vi "Create Session.vi"(8 "error in (no error)":errorcluster, 11 "Session Id":u64) -> (0 "error out":errorcluster, 1 "Run Time Configuration":string, 2 "Edit Time Configuration":string, 3 "Session out":refnum<class "Plugin Session.lvclass">, 4 "Panel Size":T1)   [LabVIEW 2021, in "InstrumentStudio Plugin SDK.lvlib" / "Plugin Session.lvclass"]
doc: "Call this VI with the Session Id as the first SDK call at the beginning of your plugin VI. This VI sets up the events and other data needed for the plugin panel and framework to communicate. If you need to know the panel size for your plugin panel to adjust its front panel, this VI will return the size. Some plugin panels support both large and small panel sizes and need to adjust the visuals on their front panel to better fit into that panel size. LabVIEW plugin panels are uniquely identified by the Plugin Session which is set by the framework when the plugin is run. Plugins must have a control named 'Session Id' which is a U64 numeric control on their plugin VI front panel so the framework can correctly set it. This 'Session Id' is then passed to Create Session.vi to begin the plugin session. This control can be placed on the user's VI by right-clicking on the input of the Create Session.vi and choosing 'Create Control'.\nThe Plugin Session returned is then used to call other SDK VIs during execution of the plugin VI to get or set properties of the plugin panel or to notify the framework of various events."
uses:
  Plugin Session.lvclass
  Panel Size.ctl
  Plugin Events.ctl
  Event Registration Refnum.ctl
  Plugin Session.lvclass/Plugin Session.ctl
  Read Edit Time Configuration.vi
  Read Run Time Configuration.vi
  InstrumentStudio Plugin SDK.lvlib
  NationalInstruments.VIHost.Interop.dll
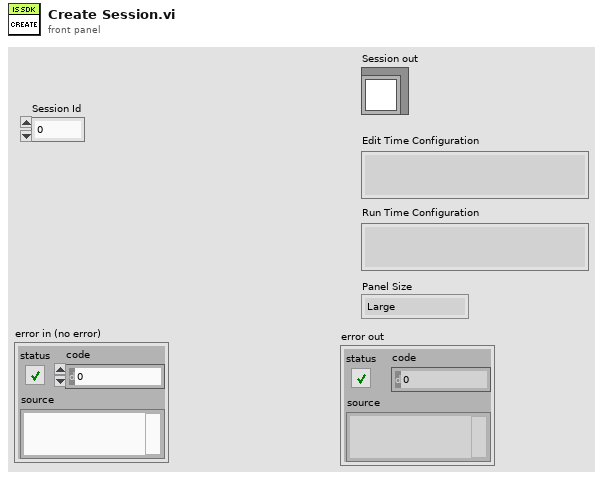
[diagram p1: front panel]
types:
  T1 = typedef "InstrumentStudio Plugin SDK.lvlib/Panel Size.ctl" = enum32{"Large", "Small"}
  T2 = typedef "InstrumentStudio Plugin SDK.lvlib/Plugin Events.ctl" = cluster{"Shutdown":refnum<user-event>, "Project Saved":refnum<user-event>, "Stop All Outputs":refnum<user-event>, "Generic Message":refnum<user-event>}
  T3 = typedef "InstrumentStudio Plugin SDK.lvlib/Event Registration Refnum.ctl" = refnum<event-registration>
  T4 = cluster{"Session Id":u64, "Plugin Events":T2, "Event Refnum":T3}
  T5 = cluster{"Name":string, "Data":string, "Completion Id":i64}
  T6 = cluster{"Project Path":path, "Completion Id":i64}
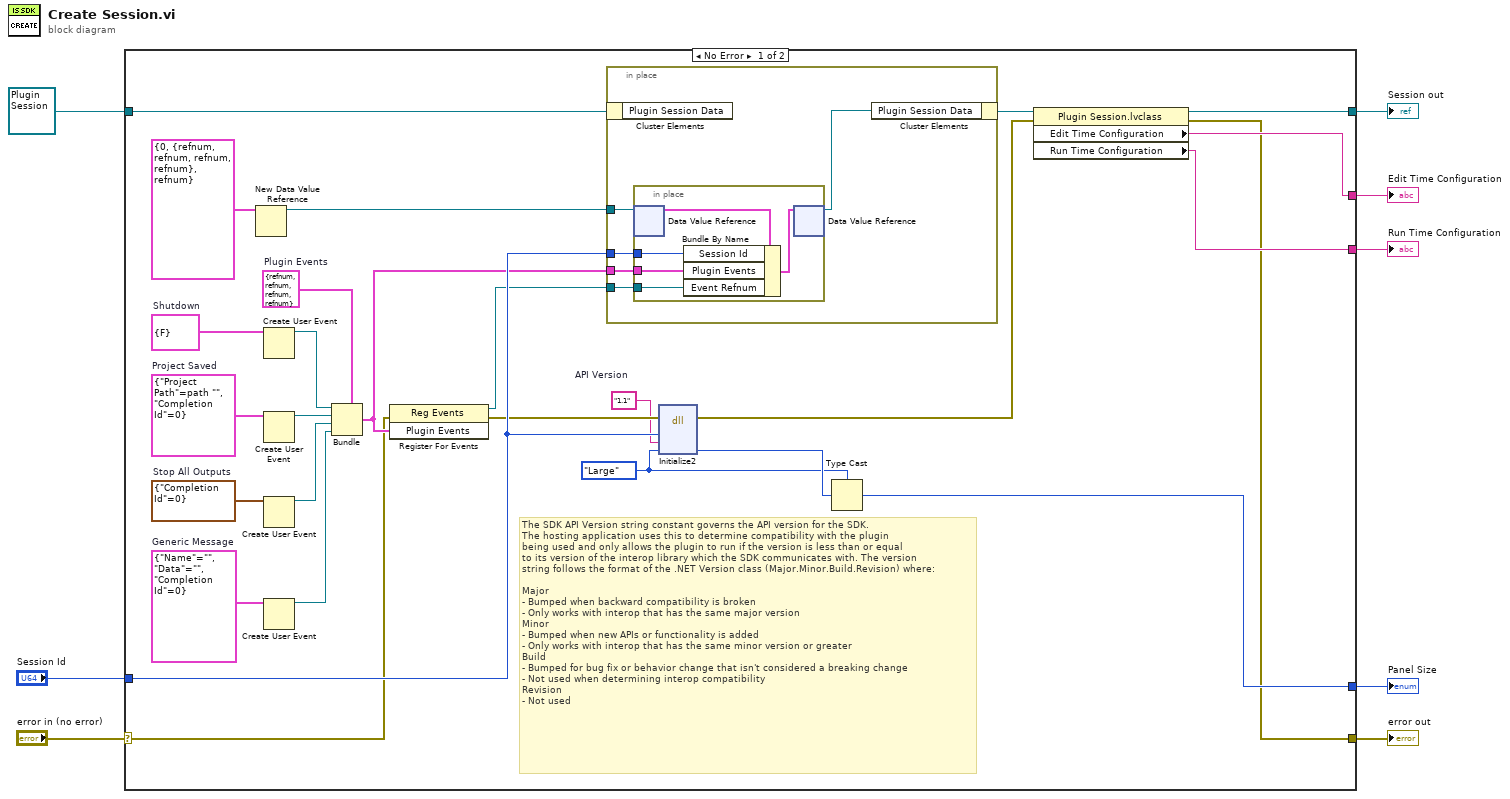
[diagram p0: block diagram]
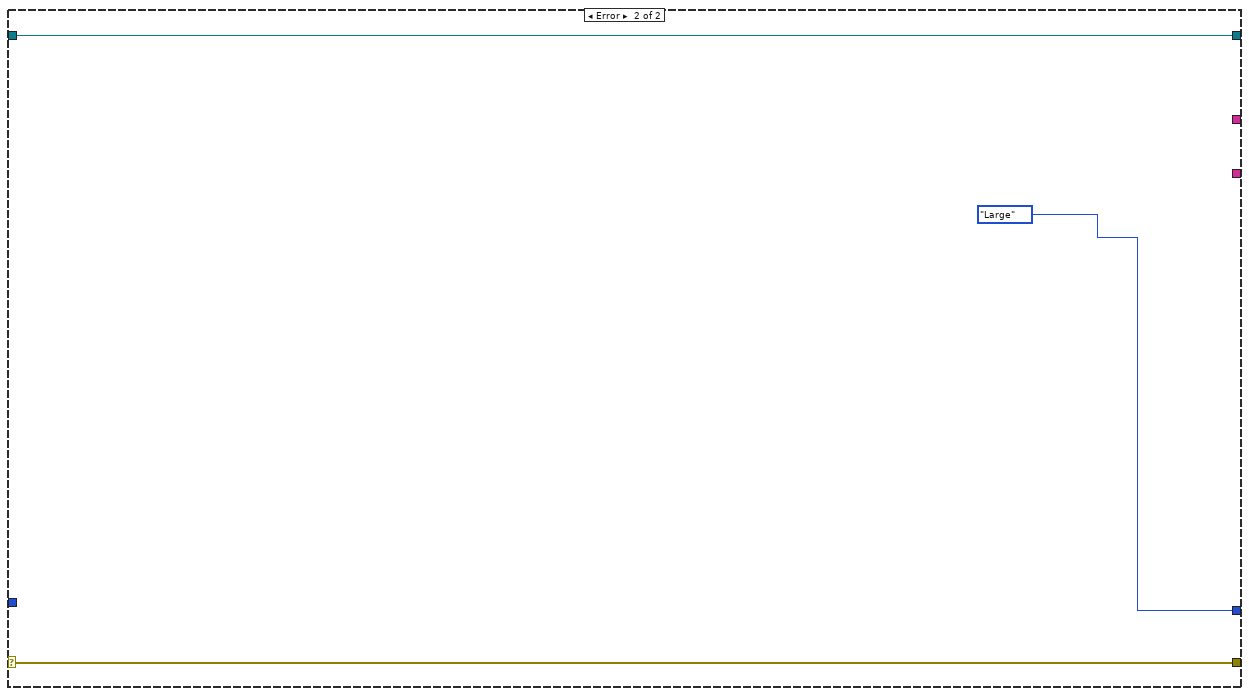
[diagram p2: hidden frame]
diagram:
  n1 = case shown="No Error" "error in (no error)" {
    selector: "error in (no error)" -> [w23 w47]
    tunnel: [w17 w47] -> w8
    tunnel: [w33 Panel_Size."Large" ("Panel Size")] -> w7
    tunnel: "Session Id" -> [w28 _]
    tunnel: refnum<class "Plugin Session.lvclass"> refnum ("PluginSDK:PluginSession.lvclass") -> [w25 w46]
    tunnel: [w18 w46] -> w3
    tunnel: [w21 _] -> w2
    tunnel: [w19 _] -> w1
    frame No Error {
      w9 = "1.1"  # API Version
      w11 = T5 {"Name"="", "Data"="", "Completion Id"=0}  # Generic Message
      w15 = cluster{"Unused":bool} {"Unused"=FALSE}  # Shutdown
      w29 = T2 {"Shutdown"=refnum, "Project Saved"=refnum, "Stop All Outputs"=refnum, "Generic Message"=refnum}  # Plugin Events
      w31 = T6 {"Project Path"=path "", "Completion Id"=0}  # Project Saved
      w32 = cluster{"Completion Id":i64} {"Completion Id"=0}  # Stop All Outputs
      w34 = Panel_Size."Large" ("Panel Size")
      # "The SDK API Version string constant governs the API version for the SDK.\nThe hosting application uses this to determine compatibility with the plugin\nbeing used and only allows the plugin to run if the version is less than or equal\nto its version of the interop library which the SDK communicates with. The version\nstring follows the format of the .NET Version class (Major.Minor.Build.Revision) where:\n\nMajor\n- Bumped when backward compatibility is broken\n- Only works with interop that has the same major version\nMinor\n- Bumped when new APIs or functionality is added\n- Only works with interop that has the same minor version or greater\nBuild\n- Bumped for bug fix or behavior change that isn't considered a breaking change\n- Not used when determining interop compatibility\nRevision\n- Not used"
      n2 = New Data Value Reference(data value=T4 {"Session Id"=0, "Plugin Events"={"Shutdown"=refnum, "Project Saved"=refnum, "Stop All Outputs"=refnum, "Generic Message"=refnum}, "Event Refnum"=refnum} ("Cluster of class private data")) -> (data value reference=w30:refnum<data-value>)  [unwired: 1 in, 1 out]
      n3 = Create User Event(user event datatype=w15) -> (user event=w14:refnum<user-event>)  [unwired: 1 in, 1 out]
      n4 = Create User Event(user event datatype=w31) -> (user event=w13:refnum<user-event>)  [unwired: 1 in, 1 out]
      n5 = Create User Event(user event datatype=w32) -> (user event=w12:refnum<user-event>)  [unwired: 1 in, 1 out]
      n6 = Create User Event(user event datatype=w11) -> (user event=w10:refnum<user-event>)  [unwired: 1 in, 1 out]
      n7 = Bundle(cluster=w29, "Shutdown"=w14, "Project Saved"=w13, "Stop All Outputs"=w12, "Generic Message"=w10) -> (w27:T2)
      n8 = register-events(error in=w23, w27) -> (reference out=w26:refnum<event-registration>, error out=w24:errorcluster)  [unwired: 1 in]
      n9 = in-place {
        in-place-border: w30 -> [w40]
        in-place-border: w28 -> [w39]
        in-place-border: w27 -> [w38]
        in-place-border: w26 -> [w37]
        n10 = in-place-cluster #1(w25) -> ()  [unwired: 1 out]
        n11 = in-place {
          in-place-border: w39 -> [w44]
          in-place-border: w38 -> [w43]
          in-place-border: w37 -> [w42]
          n12 = in-place-dvr #2(w40) -> (w45:T4)  [unwired: 1 out]
          n13 = Bundle By Name(cluster=w45, "Session Id"=w44, "Plugin Events"=w43, "Event Refnum"=w42) -> (w41:T4)
          n14 = in-place-dvr #2(w41) -> (w36:refnum<data-value>)  [unwired: 1 out]
        }
        n15 = in-place-cluster #1("Plugin Session Data"=w36) -> (w20:refnum<class "Plugin Session.lvclass">)
      }
      n16 = dll-call lib="C:/git/srd-adg-rf/dst/dstd/DSTInstStudio/source/utilities/PluginSDK/NationalInstruments.VIHost.Interop.dll" fn="Initialize2"(error in=w24, "hostId"=w28, "sdkVersion"=w9, "panelSize"=w34) -> (error out=w16:errorcluster, "panelSize"=w35:u32)  [unwired: 5 in, 1 out]
      n17 = Type Cast(type=w34, x=w35) -> (*(type *) &x=w33:T1)
      n18 = property class="Plugin Session.lvclass"(reference=w20, error in=w16) -> (reference out=w18:refnum<class "Plugin Session.lvclass">, error out=w17:errorcluster, "Edit Time Configuration"=w21:string, "Run Time Configuration"=w19:string)
    }
    frame Error {
    }
  }
  "error out" <- w8
  "Panel Size" <- w7
  "Session out" <- w3
  "Edit Time Configuration" <- w2
  "Run Time Configuration" <- w1
